vi "Edit Program.vi"() -> ()   [LabVIEW 2018]
uses:
  Subvi/Global.vi
panel:
  in  "文件管理":bool
  out "布尔":bool
  in  "Bar":bool
  in  "驱动设置":bool
  out "order":string caption="FileName:"
  out "appended path":path
  in  "编辑":bool
  in  "新建":bool
  in  "删除":bool
  in  "退出":bool
  in  "另存为":bool
  in  "保存":bool
  in  "info":bool
  out "Ready":u8(slide) max=100 scale=0.0..100.0
  in  "编辑测试项目":i32(listbox) caption="Progarm"
  out "tpdata 5":string[](array[string])
  out "子字符串之前":string
  out "tpdata 3":string[](array[string])
  out "tpdata 2":string[](array[string])
  out "Row":i32
  in  "seq":i32
  out "Copy data":string
  out "general TP info":string
  out "tpdata":string[](array[string])
  out "TP Information":string[](array[string])
  in  "Test Item":i32(listbox)
  out "Program Name:":string caption="程序名称："
  # "EditTestData"
  # "Setup"
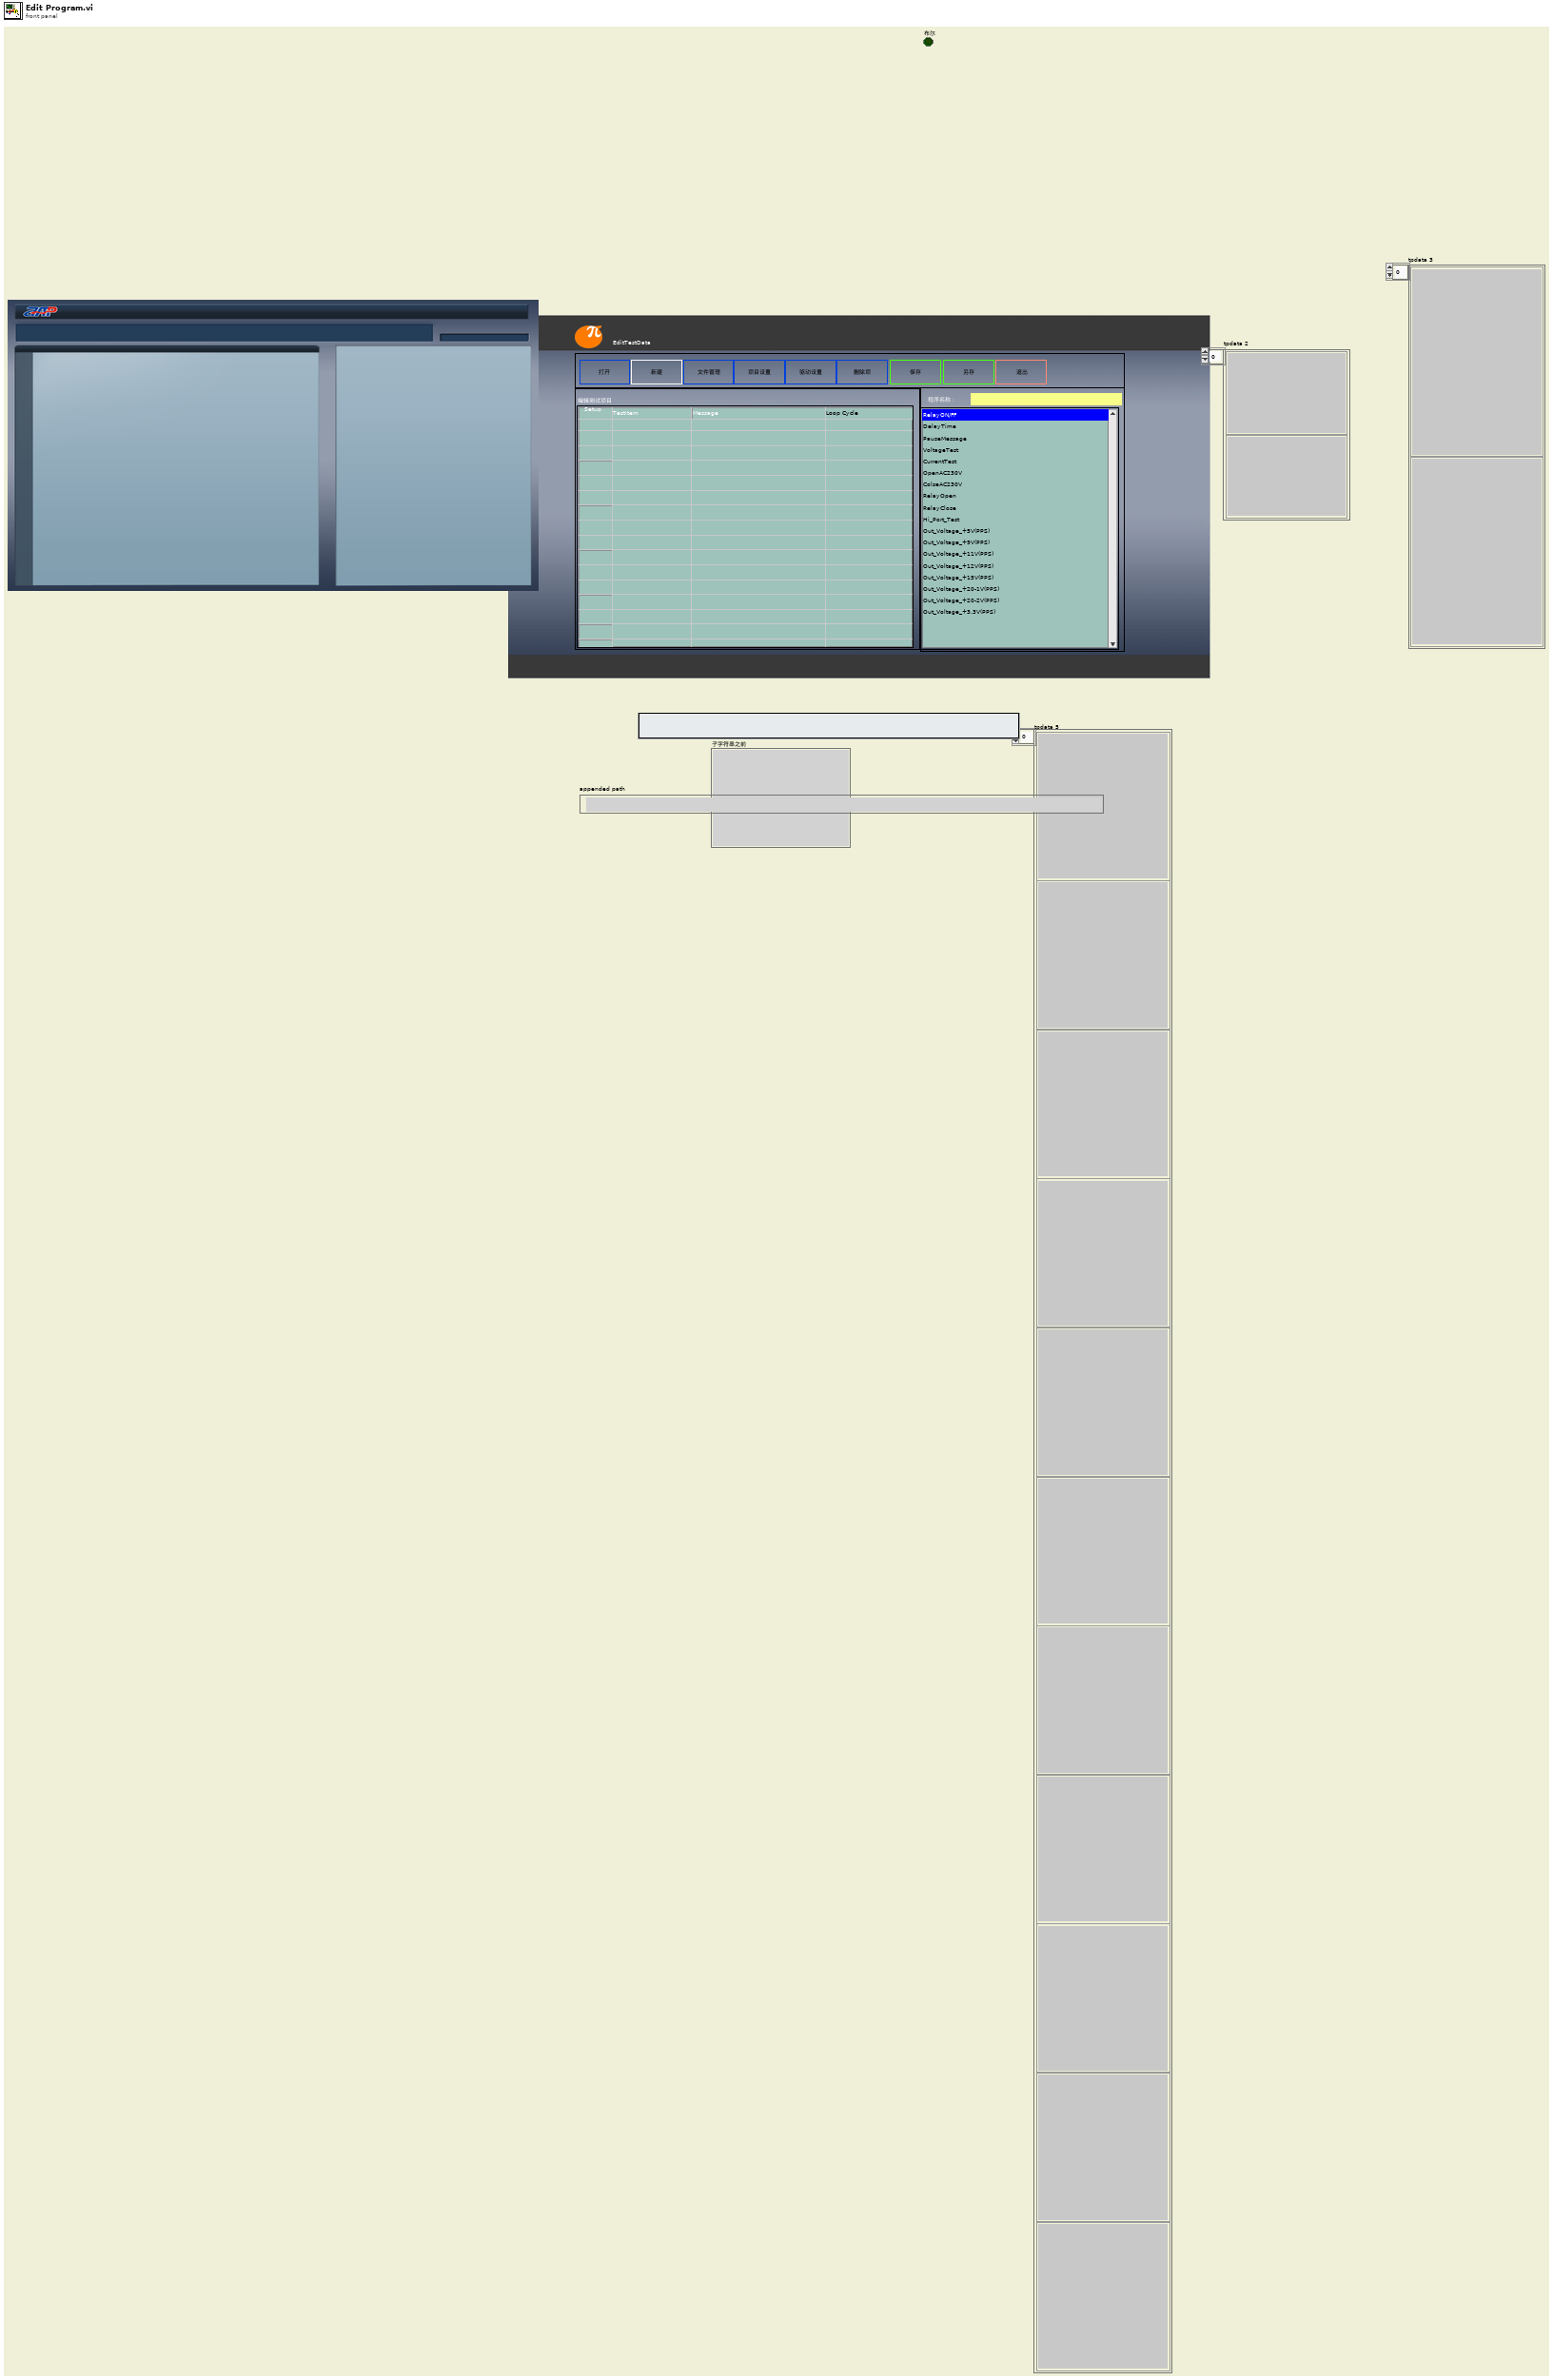
[diagram p1: front panel]
types:
  T1 = typedef "Window Refnum.ctl" = refnum<k1>
  T2 = typedef "LVPoint32TypeDef.ctl" = cluster{"Horizontal":i32, "Vertical":i32}
  T3 = typedef "LVRowAndColumnTypeDef.ctl" = cluster{"Row":i32, "Column":i32}
  T4 = typedef "Window Rectangle.ctl" = cluster{"left":i16, "top":i16, "right":i16, "bottom":i16}
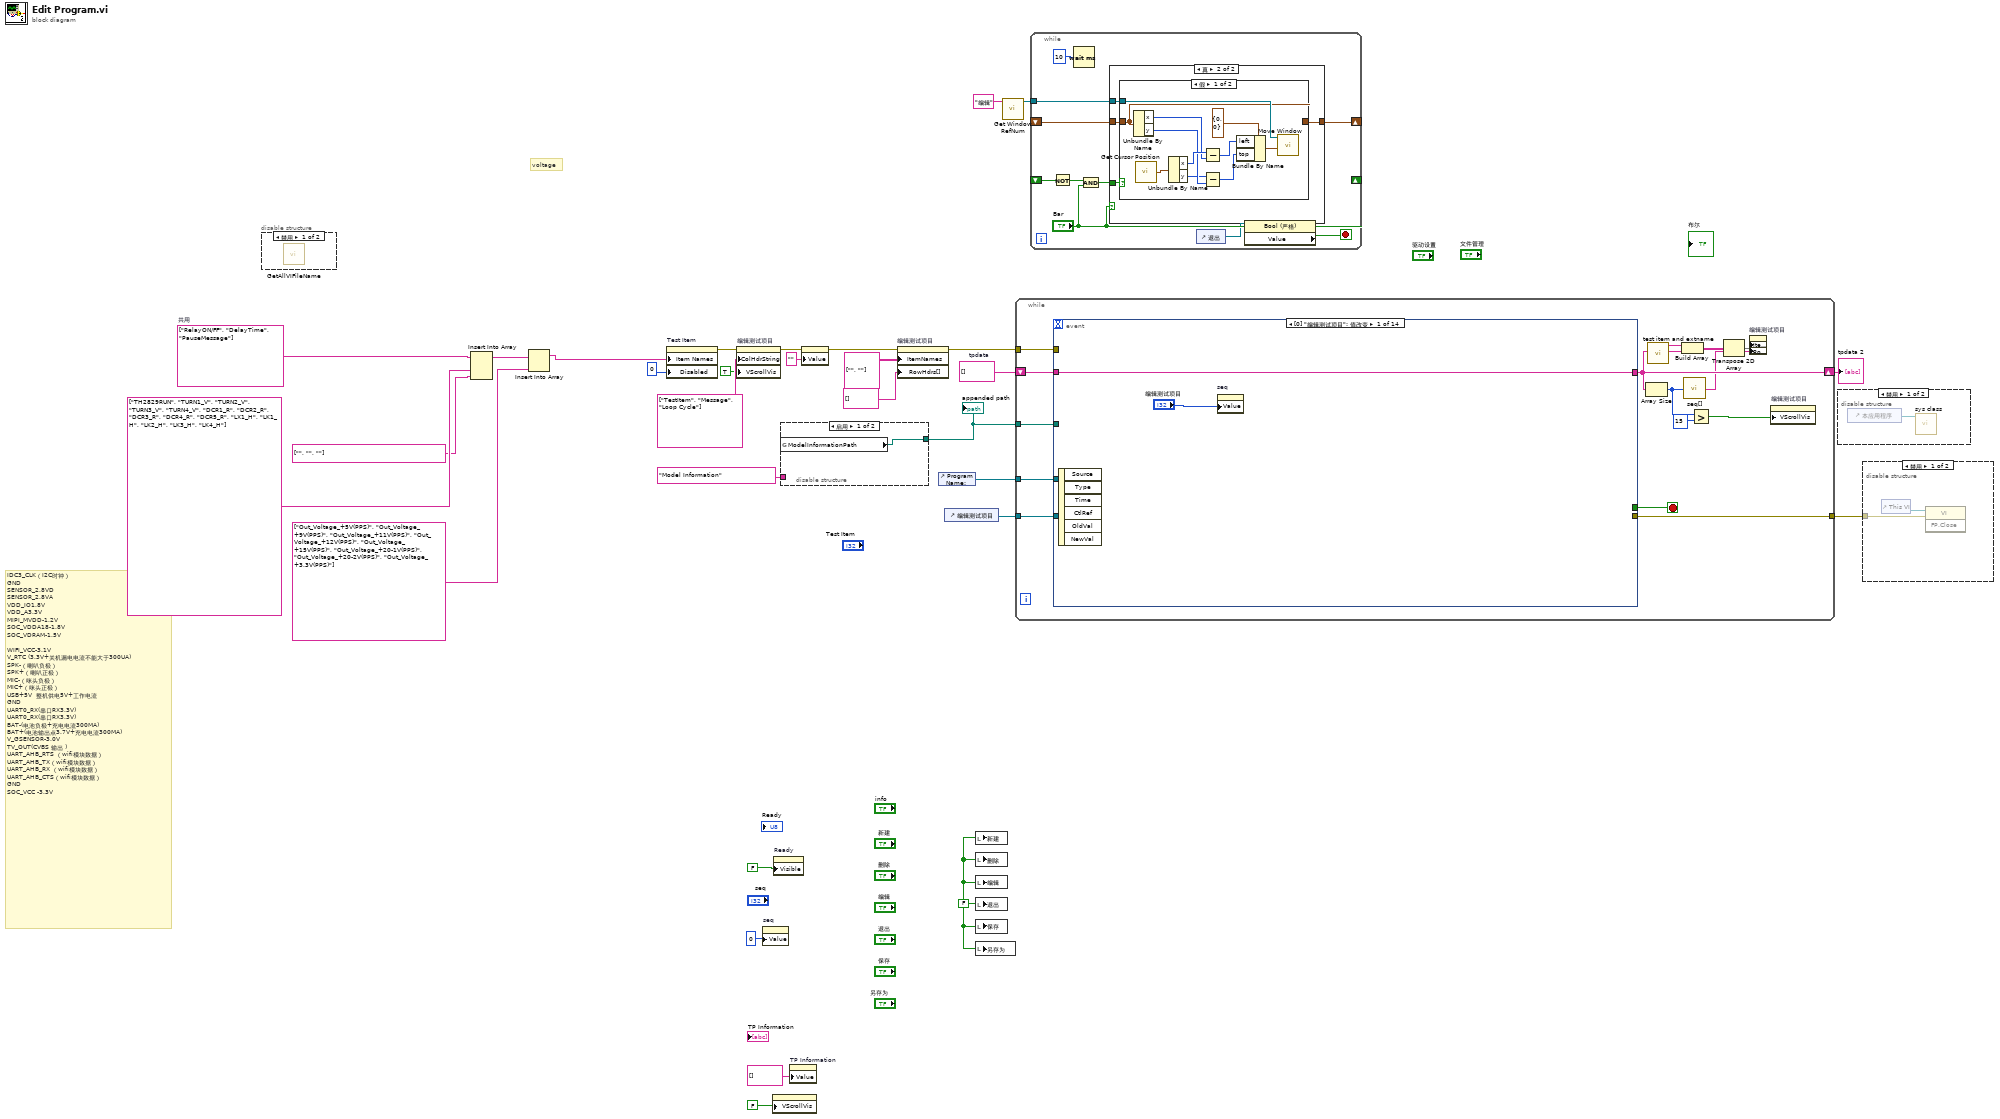
[diagram p0: block diagram]
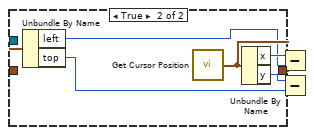
[diagram p5: hidden frame]
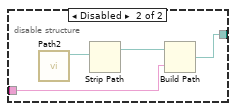
[diagram p6: hidden frame]
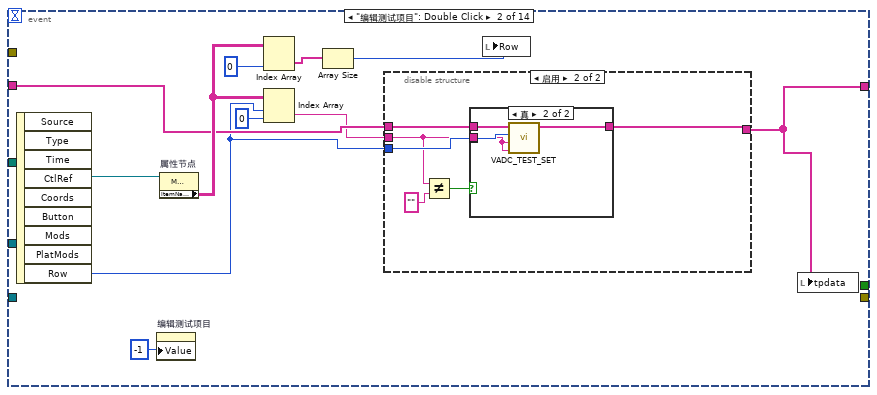
[diagram p8: hidden frame]
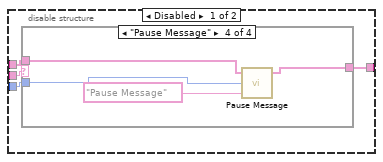
[diagram p9: hidden frame]
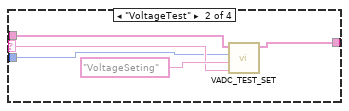
[diagram p11: hidden frame]
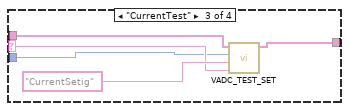
[diagram p12: hidden frame]
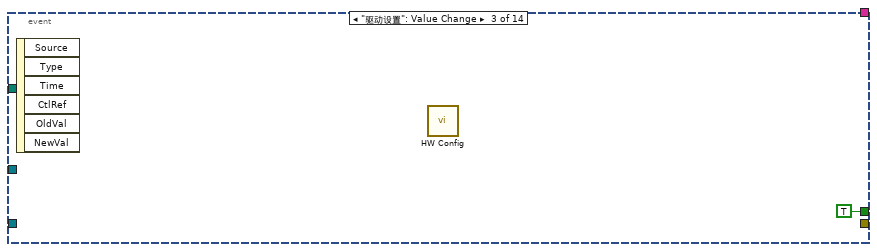
[diagram p14: hidden frame]
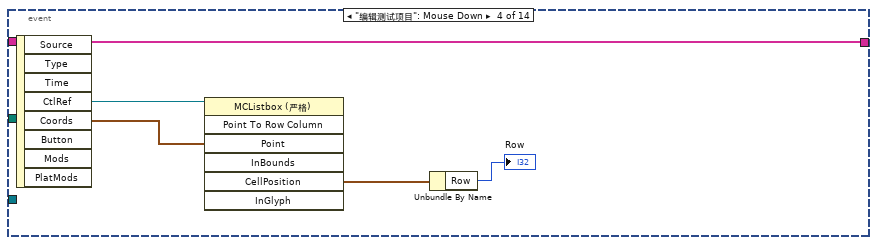
[diagram p15: hidden frame]
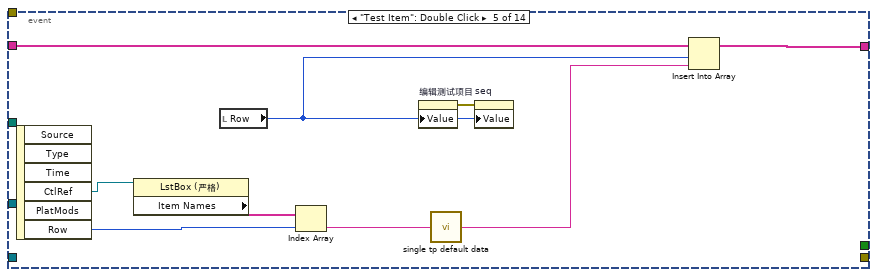
[diagram p16: hidden frame]
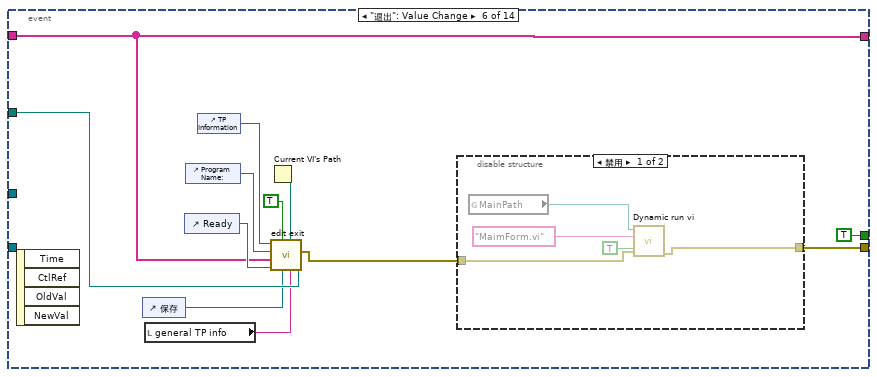
[diagram p17: hidden frame]
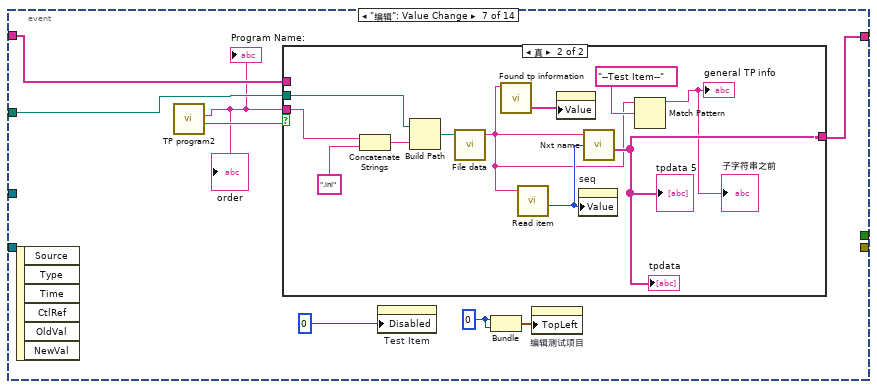
[diagram p19: hidden frame]
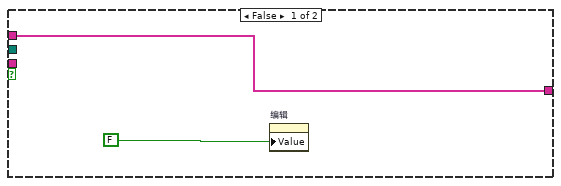
[diagram p20: hidden frame]
diagram:
  w6 = string[] ["RelayON/FF", "DelayTime", "PauseMessage"]  # 共用
  w14 = FALSE
  w21 = string[] []  # tpdata
  # "voltage"
  # "IDC3_CLK（I2C时钟）\nGND\nSENSOR_2.8VD\nSENSOR_2.8VA\nVDD_IO1.8V\nVDD_A3.3V\nMIPI_MVDD-1.2V\nSOC_VDDA18-1.8V\nSOC_VDRAM-1.5V\n \nWIFI_VCC-3.1V\nV_RTC (3.3V+关机漏电电流不能大于300UA)\nSPK-（喇叭负极）\nSPK+（喇叭正极）\nMIC-（咪头负极）\nMIC+（咪头正极）\nUSB+5V  整机供电5V+工作电流\nGND\nUART0_RX(串口RX3.3V)\nUART0_RX(串口RX3.3V)\nBAT-(电池负极+充电电流300MA)\nBAT+(电池输出点3.7V+充电电流300MA)\nV_GSENSOR-3.0V\nTV_OUT(CVBS 输出 )\nUART_AHB_RTS （wifi模块数据）\nUART_AHB_TX（wifi模块数据）\nUART_AHB_RX （wifi模块数据）\nUART_AHB_CTS（wifi模块数据）\nGND\nSOC_VCC -3.3V"
  n1 = disable-structure shown="禁用" {
    frame Disabled {
      n2 = call "GetAllVIFileName.vi"() -> ()  [unwired: 8 in, 3 out]
    }
    frame Enabled {
    }
  }
  n3 = Insert Into Array(array=w6, new element #1=string[] ["TH2829RUN", "TURN1_V", "TURN2_V", "TURN3_V", "TURN4_V", "DCR1_R", "DCR2_R", "DCR3_R", "DCR4_R", "DCR5_R", "LX1_H", "LK1_H", "LK2_H", "LK3_H", "LK4_H"], new element #2=string[] ["", "", ""]) -> (w4:string[])  [unwired: 1 in]
  n4 = Insert Into Array(array=w4, new element=string[] ["Out_Voltage_+5V(PPS)", "Out_Voltage_+9V(PPS)", "Out_Voltage_+11V(PPS)", "Out_Voltage_+12V(PPS)", "Out_Voltage_+15V(PPS)", "Out_Voltage_+20-1V(PPS)", "Out_Voltage_+20-2V(PPS)", "Out_Voltage_+3.3V(PPS)"]) -> (w3:string[])  [unwired: 1 in]
  n5 = property on="Test Item" class="LstBox (严格)"("Item Names"=w3, "Disabled"=u8 0 ("禁用")) -> (error out=w16:errorcluster)  [unwired: 2 in, 1 out]
  n6 = property on="编辑测试项目" class="MCListbox (严格)"(error in=w16, "ColHdrString"=string[] ["TestItem", "Message", "Loop Cycle"] ("Column Header Strings[]"), "VScrollVis"=TRUE ("显示项:显示垂直滚动条")) -> (error out=w17:errorcluster)  [unwired: 1 in, 1 out]
  n7 = property on="seq" class="DigNum (严格)"("Value"=0) -> ()  [unwired: 2 in, 2 out]
  n8 = property on="编辑测试项目" class="MCListbox (严格)"("VScrollVis"=FALSE ("显示项:显示垂直滚动条")) -> ()  [unwired: 2 in, 2 out]
  n9 = property on="Ready" class="Slide (严格)"("Visible"=FALSE) -> ()  [unwired: 2 in, 2 out]
  n10 = disable-structure shown="启用" {
    disable-tunnel: "Model Information" ("name or relative path") -> [_ w32]
    disable-tunnel: [w31 w33] -> w23
    frame Enabled {
      n11 = global read "Global.vi" "ModelInformationPath"() -> (w31:path)
    }
    frame Disabled {
      n12 = call "Path2.vi"() -> ("拆分的路径"=w34:path)  [unwired: 10 in, 1 out]
      n13 = Strip Path(path=w34) -> (stripped path=w35:path)  [unwired: 1 out]
      n14 = Build Path(base path=w35, name or relative path=w32) -> (appended path=w33:path)
    }
  }
  "appended path" <- w23
  n15 = property on="TP Information" class="Arr (严格)"("Value"=string[] []) -> ()  [unwired: 2 in, 2 out]
  n16 = property on="Program Name:" class="Str"(error in=w17, "Value"="") -> (error out=w29:errorcluster)  [unwired: 1 in, 1 out]
  n17 = property on="编辑测试项目" class="MCListbox (严格)"(error in=w29, "ItemNames"=string[][] [[""], [""]], "RowHdrs[]"=string[] []) -> (error out=w20:errorcluster)  [unwired: 1 in, 1 out]
  n18 = control-ref of="Program Name:"() -> (w13:refnum<vi>)
  n19 = control-ref of="编辑测试项目"() -> (w18:refnum<vi>)
  n20 = local write "新建"(w14) -> ()
  n21 = local write "删除"(w14) -> ()
  n22 = local write "编辑"(w14) -> ()
  n23 = local write "退出"(w14) -> ()
  n24 = local write "保存"(w14) -> ()
  n25 = local write "另存为"(w14) -> ()
  n26 = call "Get Window RefNum.vi"("window name (\"\")"="编辑" ("window name (\"\")")) -> ("window refnum (NaWR)"=w7:T1)  [unwired: 1 in, 7 out]
  n27 = while {
    shift-right: [w45] -> w12
    shift-left: w21 -> [w40]
    tunnel: w20 -> [w36]
    tunnel: w23 -> [w51]
    tunnel: [w49] -> w25
    tunnel: w18 -> [w46]
    tunnel: w13 -> [w37]
    stop <- w50 stop-if-true
    n28 = event shown="[0] \"编辑测试项目\": 值改变" {
      selector: _ -> [_ _ _ _ _ _ _ _ _ _ _ _ _ _]
      dyn-events: _ -> [_ _ _ _ _ _ _ _ _ _ _ _ _ _]
      timeout: _ -> [_ _ _ _ _ _ _ _ _ _ _ _ _ _]
      tunnel: [_ _ TRUE ("布尔") _ _ TRUE ("布尔") _ _ _ _ _ _ _ _] -> w50
      tunnel: w40 -> [w53 w57 _ w97 w108 w116 w134 w150 w171 w175 _ w196 w210 w214]
      tunnel: [w53 w55 _ w97 w109 w116 w135 w151 w171 w175 string[] [] ("tpdata") w194 w210 w214] -> w45
      tunnel: w51 -> [_ _ _ _ _ w121 w130 _ w169 _ w186 _ w207 w219]
      tunnel: [_ _ _ _ _ w111 _ _ _ w174 _ _ _ _] -> w49
      tunnel: w46 -> [_ _ _ _ _ _ _ _ _ _ _ w195 _ _]
      tunnel: w37 -> [_ _ _ _ _ _ _ _ w168 _ _ _ w206 _]
      tunnel: w36 -> [_ _ _ _ _ _ _ _ _ w174 _ _ _ _]
      event "编辑测试项目": Value Change {
        n29 = event-data() -> ()  [unwired: 7 out]
        n30 = property on="seq" class="DigNum (严格)"("Value"="编辑测试项目") -> ()  [unwired: 2 in, 2 out]
      }
      event "编辑测试项目": Double Click {
        n31 = event-data() -> ("CtlRef"=w63:refnum<vi>, "Row"=w56:i32)  [unwired: 8 out]
        n32 = property on="编辑测试项目" class="MCListbox (严格)"("Value"=-1 ("Progarm")) -> ()  [unwired: 2 in, 2 out]
        n33 = property on="属性节点" class="MCListbox (严格)"(reference=w63) -> ("ItemNames"=w61:string[][])  [unwired: 1 in, 2 out]
        n34 = Index Array(array=w61, index (col)=0 ("禁用的索引 (列)")) -> (element=w59:string[])  [unwired: 1 in]
        n35 = Index Array(array=w61, index (row)=w56, index (col)=0 ("disabled index (col)")) -> (element=w54:string)
        n36 = Array Size(array=w59) -> (size(s)=w58:i32)
        n37 = disable-structure shown="启用" {
          disable-tunnel: w57 -> [w68 w87]
          disable-tunnel: w56 -> [w67 w88]
          disable-tunnel: [w66 w89] -> w55
          disable-tunnel: w54 -> [w65 w85]
          frame Disabled {
            n38 = case shown="\"Pause Message\"" w65 {
              selector: w65 -> [_ w71 w76 _]
              tunnel: w68 -> [w69 w73 w78 w83]
              tunnel: [w69 w72 w77 w82] -> w66
              tunnel: w67 -> [_ w70 w75 w81]
              frame "0", Default {
              }
              frame "VoltageTest" {
                n39 = call "VADC_TEST_SET.vi"("itemiput"=w71, "input"="VoltageSeting" ("字符串"), "SEQ"=w70, "tpdata in"=w73) -> ("tpdata out"=w72:string[])  [unwired: 3 in]
              }
              frame "CurrentTest" {
                n40 = call "VADC_TEST_SET.vi"("itemiput"=w76, "input"="CurrentSetig" ("字符串"), "SEQ"=w75, "tpdata in"=w78) -> ("tpdata out"=w77:string[])  [unwired: 3 in]
              }
              frame "Pause Message" {
                n41 = call "Pause Message.vi"("字符串"="Pause Message", "SEQ"=w81, "tpdata"=w83) -> ("ta data out"=w82:string[])  [unwired: 2 in]
              }
            }
          }
          frame Enabled {
            n42 = Not Equal?(x=w85, y="") -> (x != y?=w84:bool)
            n43 = case shown="真" w84 {
              tunnel: [w90 w94] -> w89
              tunnel: w88 -> [_ w93]
              tunnel: w87 -> [w90 w92]
              tunnel: w85 -> [_ w91]
              frame False {
              }
              frame True {
                n44 = call "VADC_TEST_SET.vi"("itemiput"=w91, "input"=w91, "SEQ"=w93, "tpdata in"=w92) -> ("tpdata out"=w94:string[])  [unwired: 3 in]
              }
            }
          }
        }
        n45 = local write "Row"(w58) -> ()
        n46 = local write "tpdata"(w55) -> ()
      }
      event "驱动设置": Value Change {
        n47 = event-data() -> ()  [unwired: 7 out]
        n48 = call "HW Config.vi"() -> ()  [unwired: 1 in]
      }
      event "编辑测试项目": Mouse Down {
        n49 = event-data() -> ("CtlRef"=w96:refnum<vi>, "Coords"=w100:T2)  [unwired: 7 out]
        n50 = invoke class="MCListbox (严格)" method="Point To Row Column"(reference=w96, "Point"=w100) -> ("CellPosition"=w99:T3)  [unwired: 5 in, 6 out]
        n51 = Unbundle By Name(w99) -> ("Row"=→"Row":i32)
      }
      event "Test Item": Double Click {
        n52 = event-data() -> ("CtlRef"=w105:refnum<vi>, "Row"=w107:i32)  [unwired: 5 out]
        n53 = property on="属性节点" class="LstBox (严格)"(reference=w105) -> ("Item Names"=w102:string[])  [unwired: 1 in, 2 out]
        n54 = local read "Row"() -> (w101:i32)
        n55 = Index Array(array=w102, index=w107) -> (element=w104:string)
        n56 = property on="编辑测试项目" class="MCListbox (严格)"("Value"=w101) -> (error out=w106:errorcluster)  [unwired: 2 in, 1 out]
        n57 = call "single tp default data.vi"("字符串"=w104) -> ("item data"=w103:string)
        n58 = property on="seq" class="DigNum (严格)"(error in=w106, "Value"=w101) -> ()  [unwired: 1 in, 2 out]
        n59 = Insert Into Array(array=w108, index=w101, new element=w103) -> (w109:string[])
      }
      event "退出": Value Change {
        n60 = event-data() -> ()  [unwired: 5 out]
        n61 = control-ref of="保存"() -> (w117:refnum<vi>)
        n62 = local read "general TP info"() -> (w115:string)
        n63 = control-ref of="Ready"() -> (w118:refnum<vi>)
        n64 = control-ref of="Program Name:"() -> (w119:refnum<vi>)
        n65 = control-ref of="TP Information"() -> (w120:refnum<vi>)
        n66 = Current VI's Path() -> (path=w114:path)
        n67 = call "edit exit.vi"("appended path"=w121, "genneral info"=w115, "path"=w114, "保存"=w117, "Edit"=TRUE, "Ready"=w118, "tpdata"=w116, "Program Name:"=w119, "TP Information"=w120) -> ("error out"=w112:errorcluster)  [unwired: 1 in, 1 out]
        n68 = disable-structure shown="禁用" {
          disable-tunnel: w112 -> [w123 w127]
          disable-tunnel: [w122 w127] -> w111
          frame Disabled {
            n69 = global read "Global.vi" "MainPath"() -> (w126:path)
            n70 = call "Dynamic run vi.vi"("error in (no error)"=w123, "Wait Until Done"=TRUE, "vi name"="MaimForm.vi", "path"=w126) -> ("error out"=w122:errorcluster)  [unwired: 4 out]
          }
          frame Enabled {
          }
        }
      }
      event "编辑": Value Change {
        w132 = 0
        n71 = event-data() -> ()  [unwired: 7 out]
        n72 = call "TP program2.vi"() -> ("布尔 2"=w129:bool, "order"=w128:string)  [unwired: 10 in]
        "order" <- w128
        "Program Name:" <- w128
        n73 = case shown="真" w129 {
          tunnel: w130 -> [_ w147]
          tunnel: w128 -> [_ w144]
          tunnel: [w137 w142] -> w135
          tunnel: w134 -> [w137 _]
          frame False {
            n74 = property on="编辑" class="Bool (严格)"("Value"=FALSE) -> ()  [unwired: 2 in, 2 out]
          }
          frame True {
            n75 = Concatenate Strings(w144, ".ini") -> (w145:string)
            n76 = Build Path(base path=w147, name or relative path=w145) -> (appended path=w148:path)
            n77 = call "File data.vi"("file path (use dialog)"=w148) -> ("File data"=w139:string)  [unwired: 1 in, 3 out]
            n78 = call "Found tp information.vi"("TP DATA"=w139) -> ("TP Information(array)"=w143:string[])  [unwired: 10 out]
            n79 = call "Read item.vi"("data in"=w139) -> ("Seq numbers"=w141:i32)  [unwired: 1 in, 4 out]
            n80 = property on="TP Information" class="Arr (严格)"("Value"=w143) -> ()  [unwired: 2 in, 2 out]
            n81 = property on="seq" class="DigNum (严格)"("Value"=w141) -> ()  [unwired: 2 in, 2 out]
            n82 = call "Nxt name.vi"("Full string"=w139, "MAX"=w141) -> ("tpdata"=w142:string[])  [unwired: 1 in, 3 out]
            "tpdata" <- w142
            "tpdata 5" <- w142
            n83 = Match Pattern(string=w139, regular expression="--Test Item--") -> (before substring=→"general TP info" →"子字符串之前":string)  [unwired: 4 out]
          }
        }
        n84 = property on="Test Item" class="LstBox (严格)"("Disabled"=u8 0 ("禁用")) -> ()  [unwired: 2 in, 2 out]
        n85 = Bundle(w132, w132) -> (w131:cluster{i32, i32})  [unwired: 1 out]
        n86 = property on="编辑测试项目" class="MCListbox (严格)"("TopLeft"=w131) -> ()  [unwired: 2 in, 2 out]
      }
      event "编辑测试项目": Shortcut Menu Selection (User) {
        n87 = event-data() -> ("ItemPath"=w152:string)  [unwired: 8 out]
        n88 = property on="Row" class="DigNum (严格)"() -> ("Value"=w149:i32)  [unwired: 2 in, 2 out]
        n89 = case shown="\"粘贴该测试项目\"" w152 {
          tunnel: [w153 w161] -> w151
          tunnel: w150 -> [w153 w156]
          tunnel: w149 -> [w154 w160]
          frame "复制该测试项目", Default {
            n90 = Index Array(array=w153, index=w154) -> (element=→"Copy data":string)
          }
          frame "粘贴该测试项目" {
            n91 = local read "Copy data"() -> (w158:string)
            n92 = Not Equal?(x=w158, y="") -> (x != y?=w159:bool)
            n93 = case shown="真" w159 {
              tunnel: [w162 w165] -> w161
              tunnel: w158 -> [_ w167]
              tunnel: w160 -> [_ w166]
              tunnel: w156 -> [w162 w163]
              frame False {
              }
              frame True {
                n94 = Insert Into Array(array=w163, index=w166, new element=w167) -> (w165:string[])
                n95 = Array Size(array=w165) -> (size(s)=w164:i32)
                n96 = property on="seq" class="DigNum (严格)"("Value"=w164) -> ()  [unwired: 2 in, 2 out]
              }
            }
          }
        }
      }
      event "另存为": Value Change {
        n97 = event-data() -> ()  [unwired: 7 out]
        n98 = control-ref of="另存为"() -> (w173:refnum<vi>)
        n99 = control-ref of="Ready"() -> (w172:refnum<vi>)
        n100 = local read "general TP info"() -> (w170:string)
        n101 = call "edit save as.vi"("genneral info"=w170, "tpdata"=w171, "appended path"=w169, "Slide引用句柄"=w172, "filename"=w168, "Bool引用句柄"=w173) -> ()  [unwired: 2 in]
      }
      event "文件管理": Value Change {
        n102 = event-data() -> ()  [unwired: 7 out]
        n103 = call "FileAdministrotar.vi"() -> ()  [unwired: 12 in]
      }
      event "新建": Value Change {
        n104 = event-data() -> ()  [unwired: 7 out]
        n105 = Strip Path(path=w186) -> (stripped path=w184:path)  [unwired: 1 out]
        n106 = Build Path(base path=w184, name or relative path="HW Config File") -> (appended path=w181:path)
        n107 = property on="Program Name:" class="Str"("Value"="") -> ()  [unwired: 2 in, 2 out]
        n108 = call "TP Information.vi"("TP information in"=string[] [], "base path"=w181) -> ("TP Information out"=w177:string[])  [unwired: 9 out]
        n109 = property on="TP Information" class="Arr (严格)"("Value"=w177) -> (error out=w178:errorcluster)  [unwired: 2 in, 1 out]
        n110 = call "array to general.vi"("TP Information out"=w177) -> ("字符串"=w176:string)
        n111 = local write "general TP info"(w176) -> ()
        n112 = property on="Test Item" class="LstBox (严格)"(error in=w178, "Disabled"=u8 0 ("禁用")) -> ()  [unwired: 1 in, 2 out]
      }
      event "删除": Value Change {
        w192 = u16 4 items=["OK", "OK+Cancel", "Abort+Retry+Ignore", "Yes+ON+Cancel", "Yes+No", "Retry+Cancel", "Cancel+Retry+Continue"] ("Buttons")
        w193 = u16 2 items=["None", "Critical", "Question", "Exclamation", "Infomation"] ("Icon")
        n113 = event-data() -> ()  [unwired: 7 out]
        n114 = call "user32.vi"("Icon"=w193, "Buttons"=w192, "Ipcaption"="TP Editor", "IP Text"="您确定要删除此项目？") -> ("buttin pressed"=w190:i32)  [unwired: 1 out]
        n115 = Equal?(x=w190, y=6) -> (x = y?=w188:bool)
        n116 = case shown="假" w188 {
          tunnel: w196 -> [w198 w204]
          tunnel: w195 -> [_ w203]
          tunnel: [w198 w200] -> w194
          tunnel: [FALSE TRUE] -> _
          frame False {
          }
          frame True {
            n117 = property class="MCListbox (严格)"(reference=w203) -> ("Value"=w202:i32)  [unwired: 1 in, 2 out]
            n118 = Delete From Array(array=w204, length=1 ("长度"), index=w202) -> (array with subset deleted=w200:string[])  [unwired: 1 out]
          }
        }
      }
      event "保存": Value Change {
        n119 = event-data() -> ()  [unwired: 7 out]
        n120 = local read "general TP info"() -> (w209:string)
        n121 = control-ref of="Ready"() -> (w208:refnum<vi>)
        n122 = call "edit save.vi"("Slide"=w208, "appended path"=w207, "filename"=w206, "edit"=TRUE, "genneral info"=w209, "tpdata"=w210) -> ()  [unwired: 5 out]
        "tpdata 3" <- w210
      }
      event "info": Value Change {
        n123 = event-data() -> ()  [unwired: 7 out]
        n124 = Strip Path(path=w219) -> (stripped path=w218:path)  [unwired: 1 out]
        n125 = property on="Program Name:" class="Str"() -> ("Value"=w212:string)  [unwired: 2 in, 2 out]
        n126 = Not Equal?(x=w212, y="") -> (x != y?=w211:bool)
        n127 = Build Path(base path=w218, name or relative path="HW Config File") -> (appended path=w217:path)
        n128 = property on="TP Information" class="Arr (严格)"() -> ("Value"=w215:string[])  [unwired: 2 in, 2 out]
        n129 = case shown="真" w211 {
          tunnel: w217 -> [_ w226]
          tunnel: w215 -> [_ w225]
          frame False {
            n130 = One Button Dialog(message="程序名称不能为空，请选择后重试" ("消息")) -> ()  [unwired: 1 in, 1 out]
          }
          frame True {
            n131 = call "TP Information.vi"("TP information in"=w225, "base path"=w226) -> ("TP Information out"=w222:string[])  [unwired: 9 out]
            n132 = Equal?(x=w222, y=w225) -> (x = y?=w224:bool[])
            n133 = call "array to general.vi"("TP Information out"=w222) -> ("字符串"=w221:string)
            n134 = And Array Elements(Boolean array=w224) -> (logical AND=w223:bool)
            n135 = property on="TP Information" class="Arr (严格)"("Value"=w222) -> ()  [unwired: 2 in, 2 out]
            n136 = Not(x=w223) -> ()  [unwired: 1 out]
            n137 = local write "general TP info"(w221) -> ()
          }
        }
      }
    }
    n138 = Array Size(array=w45) -> (size(s)=w42:i32)
    n139 = call "test item and extname.vi"("tpdata"=w45) -> ("Nxt.Name"=w43:string[], "test item"=w44:string[])  [unwired: 9 out]
    n140 = Build Array(w44, w43) -> (w41:string[][])
    n141 = call "seq[].vi"("数值"=w42) -> ("数组"=w38:string[])
    n142 = Greater?(x=w42, y=15) -> (0:w47:bool)
    n143 = Transpose 2D Array(2D array=w41) -> (transposed array=w39:string[][])
    n144 = property on="编辑测试项目" class="MCListbox (严格)"("ItemNames"=w39, "RowHdrs[]"=w38) -> ()  [unwired: 2 in, 2 out]
    n145 = property on="编辑测试项目" class="MCListbox (严格)"("VScrollVis"=w47) -> ()  [unwired: 2 in, 2 out]
  }
  "tpdata 2" <- w12
  n146 = while {
    shift-left: _ -> [w230]
    shift-right: [w231] -> _
    shift-left: _ -> [w234]
    shift-right: ["Bar"] -> _
    tunnel: w7 -> [w235]
    stop <- w228 stop-if-true
    n147 = Not(x=w234) -> (.not. x?=w233:bool)
    n148 = Wait (ms)(milliseconds to wait=u32 10) -> ()  [unwired: 1 out]
    n149 = And(x=w233, y="Bar") -> (x .and. y?=w229:bool)
    n150 = case shown="真" "Bar" {
      tunnel: w235 -> [_ w241]
      tunnel: [w237 w240] -> w231
      tunnel: w230 -> [w237 w238]
      tunnel: w229 -> [_ w239]
      frame False {
      }
      frame True {
        n151 = case shown="假" w239 {
          tunnel: w241 -> [w247 w263]
          tunnel: [w242 w253] -> w240
          tunnel: w238 -> [w242 _]
          frame False {
            n152 = Unbundle By Name(w242) -> ("x"=w250:i16, "y"=w249:i16)
            n153 = call "Get Cursor Position.vi"() -> ("cursor position"=w252:cluster{"x":i16, "y":i16})
            n154 = Unbundle By Name(w252) -> ("x"=w251:i16, "y"=w248:i16)
            n155 = Subtract(x=w251, y=w250) -> (x-y=w244:i16)
            n156 = Subtract(x=w248, y=w249) -> (x-y=w245:i16)
            n157 = Bundle By Name(cluster=cluster{"left":i16, "top":i16} {"left"=0, "top"=0} ("new position (0,0)"), "left"=w244, "top"=w245) -> (w243:cluster{"left":i16, "top":i16})
            n158 = call "Move Window.vi"("new position (0,0)"=w243, "window refnum (NaWR)"=w247) -> ()  [unwired: 2 in, 4 out]
          }
          frame True {
            n159 = call "Get Window Rectangle.vi"("window refnum (NaWR)"=w263) -> ("window rect"=w262:T4)  [unwired: 1 in, 5 out]
            n160 = call "Extract Window Origin.vi"("window rect"=w262) -> ("window origin"=w261:cluster{"left":i16, "top":i16})  [unwired: 1 out]
            n161 = Unbundle By Name(w261) -> ("left"=w258:i16, "top"=w257:i16)
            n162 = call "Get Cursor Position.vi"() -> ("cursor position"=w260:cluster{"x":i16, "y":i16})
            n163 = Unbundle By Name(w260) -> ("x"=w259:i16, "y"=w256:i16)
            n164 = Subtract(x=w259, y=w258) -> (x-y=w254:i16)
            n165 = Subtract(x=w256, y=w257) -> (x-y=w255:i16)
            n166 = Bundle By Name(cluster=w260, "x"=w254, "y"=w255) -> (w253:cluster{"x":i16, "y":i16})
          }
        }
      }
    }
    n167 = control-ref of="退出"() -> (w227:refnum<vi>)
    n168 = property on="属性节点" class="Bool (严格)"(reference=w227) -> ("Value"=w228:bool)  [unwired: 1 in, 2 out]
  }
  n169 = disable-structure shown="禁用" {
    frame Disabled {
      n170 = control-ref of="本应用程序"() -> (w264:refnum<vi>)
      n171 = call "sys class.vi"("应用程序输入"=w264) -> ()  [unwired: 9 in, 2 out]
    }
    frame Enabled {
    }
  }
  n172 = disable-structure shown="禁用" {
    disable-tunnel: w25 -> [w266 _]
    frame Disabled {
      n173 = control-ref of="This VI"() -> (w265:refnum<vi>)
      n174 = invoke class="VI" method="FP.Close"(reference=w265, error in=w266) -> ()  [unwired: 1 in, 3 out]
    }
    frame Enabled {
    }
  }
